vi "LVClass_HasoEngine Set AlgoType.vi"(0 "HasoEngine in":refnum<class "HasoEngine.lvclass">, 5 "Algorithm":T1, 11 "error in (no error)":errorcluster) -> (4 "HasoEngine out":refnum<class "HasoEngine.lvclass">, 15 "error out":errorcluster)   [LabVIEW 2020, in "HasoEngine.lvclass"]
doc: "Spots detection algorithm type setter.\n\n--------------------------------------------------------------------------------\n\n<B>HasoEngineIn </B> : HasoEngine object.\n<B>HasoEngineOut </B> : HasoEngine object.\n<B>algo_type </B> : Spots detection algorithm type : standard (0) or fast (1).\n<B>ErrorIn </B> : Error\n<B>ErrorOut </B> : Error\n\n--------------------------------------------------------------------------------"
uses:
  HasoEngine.lvclass
  Controls/Algo choice.ctl
  HasoEngine.lvclass/HasoEngine.ctl
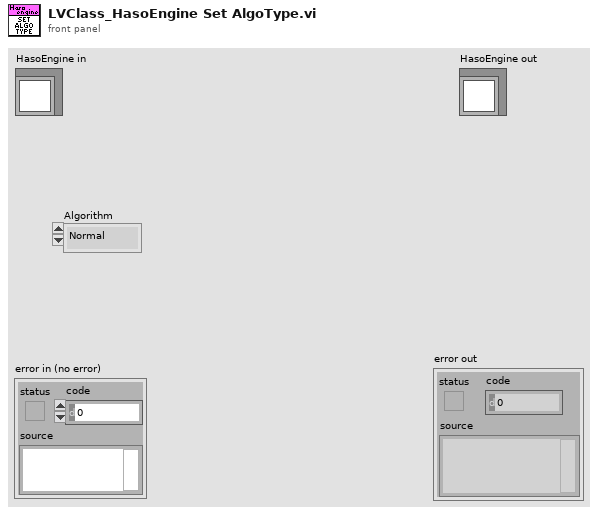
[diagram p1: front panel]
types:
  T1 = typedef "Algo choice.ctl" = enum16{"Normal", "Fast"}
  T2 = typedef "ClassID.ctl" = i64
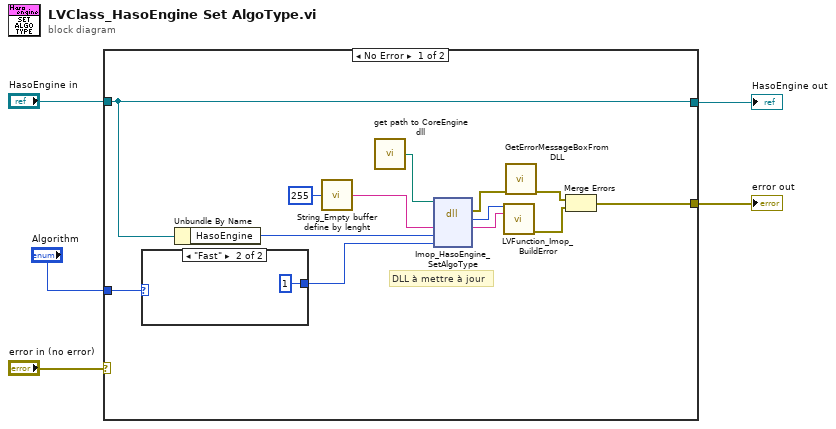
[diagram p0: block diagram]
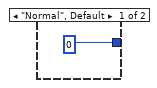
[diagram p2: hidden frame]
diagram:
  n1 = case shown="No Error" "error in (no error)" {
    selector: "error in (no error)" -> [_ w21]
    tunnel: "HasoEngine in" -> [w13 w22]
    tunnel: [w13 w22] -> w2
    tunnel: [w8 w21] -> w3
    tunnel: "Algorithm" -> [w6 _]
    frame No Error {
      # "DLL à mettre à jour"
      n2 = case shown="\"Fast\"" w6 {
        tunnel: [0 ("algo_type") 1 ("algo_type")] -> w7
        frame "Normal", Default {
        }
        frame "Fast" {
        }
      }
      n3 = Unbundle By Name(w13) -> ("HasoEngine"=w12:T2)
      n4 = call "String_Empty buffer define by lenght.vi"("Lenght (255)"=255) -> ("Empty buffer"=w16:string)
      n5 = call "get path to CoreEngine dll.vi"() -> ("path to wavekit library"=w15:path)  [unwired: 14 in, 1 out]
      n6 = dll-call lib="D:/soft/HASO_v3/SVN_trunk/ImOpCoreEngine4_LV2011/DLLs/c_interface_vc100.dll" fn="Imop_HasoEngine_SetAlgoType"(path in=w15, "message"=w16, "hasoEngine"=w12, "algo_type"=w7) -> (error out=w14:errorcluster, "return type"=w17:i32, "message"=w18:string)  [unwired: 4 in, 1 out]
      n7 = call "LVFunction_Imop_BuildError.vi"("code"=w17, "String to Prepend to source (\"\")"=w18) -> ("error out"=w9:errorcluster)  [unwired: 13 in]
      n8 = call "GetErrorMessageBoxFromDLL.vi"("error IN"=w14) -> ("error OUT"=w10:errorcluster)  [unwired: 10 in]
      n9 = Merge Errors(w10, w9) -> (w8:errorcluster)
    }
    frame Error {
    }
  }
  "error out" <- w3
  "HasoEngine out" <- w2
